vi "Module Top Level.vi"(8 "error in":errorcluster, 11 "Chassis3FPGA":T1) -> (0 "error out":errorcluster)   [LabVIEW 2018, in "ARINC.lvlib"]
doc: "This is the top level VI for this module. It uses a queue for communications and is stopped user a user event. The general architecture is similar to a simple queued message handler.\n\nThe VIs associated with this module are organized in a LabVIEW Library."
uses:
  ARINC.lvlib
  FPGA/Chassis3FPGARef.ctl
  Private Controls/Host Comms Data.ctl
  Private Controls/Module Data.ctl
  Private Controls/Module Action.ctl
  <vilib>/Utility/error.llb/Error Cluster From Error Code.vi
  <vilib>/rvi/errors/niLvFpgaAdjustHostInterfaceError.vi
  <vilib>/rvi/interface/nirviMethod/nirviMethod.xnode
  <vilib>/rvi/interface/nirviReadWriteControl/nirviReadWriteControl.xnode
  RT-UDP Writer/UDP Writer.lvlib
  <vilib>/FPGAPlugInAG/Dynamic/niLvFpga_AcknowledgeIrq_Dynamic.vi
  NiFpgaLv.dll
  <vilib>/rvi/interface/Simulation/niFpgaSimulationCallBeginRW.vi
  <vilib>/FPGAPlugInAG/Dynamic/niLvFpga_StartFifo_Dynamic.vi
  <vilib>/rvi/errors/niLvFpgaMergeErrorWithErrorCode.vi
panel:
  out "Data":u32[](array[numeric])
  # "ARINC"
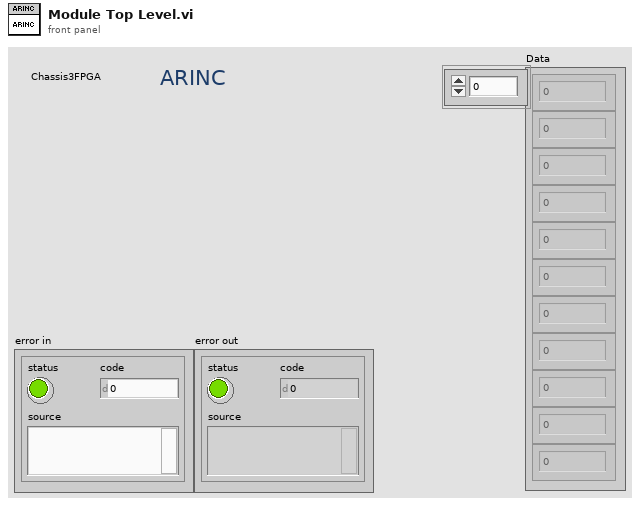
[diagram p1: front panel]
types:
  T1 = typedef "Chassis3FPGARef.ctl" = refnum<k20>
  T2 = typedef "ARINC.lvlib/Host Comms Data.ctl" = cluster{"Connected?":bool, "Arinc Data":sgl[]}
  T3 = typedef "ARINC.lvlib/Module Data.ctl" = cluster{"Data":variant, "Action":T4}
  T4 = typedef "ARINC.lvlib/Module Action.ctl" = enum16{"Init", "Write(Tx)", "Read(Rx)", "Error"}
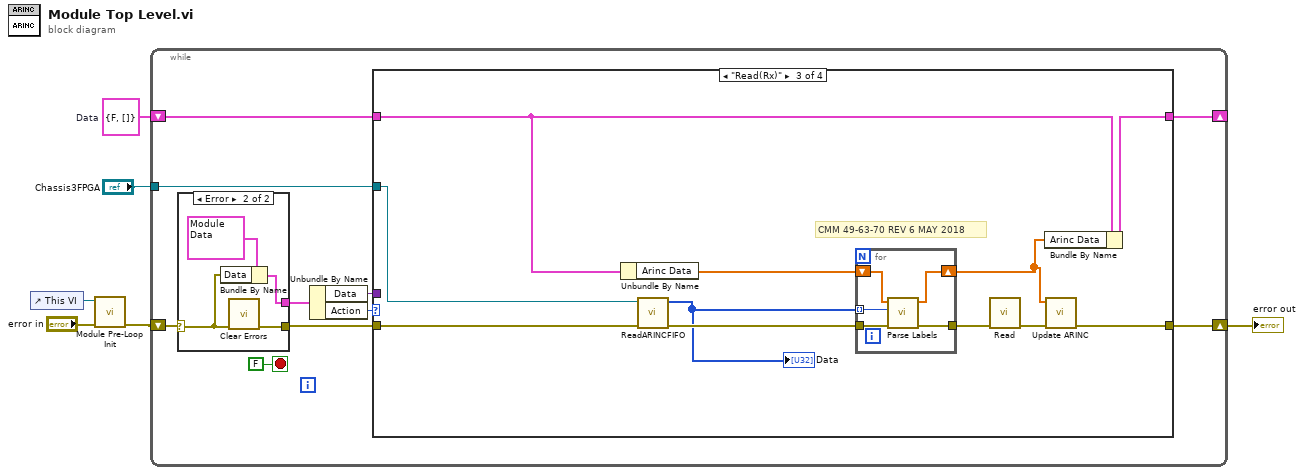
[diagram p0: block diagram]
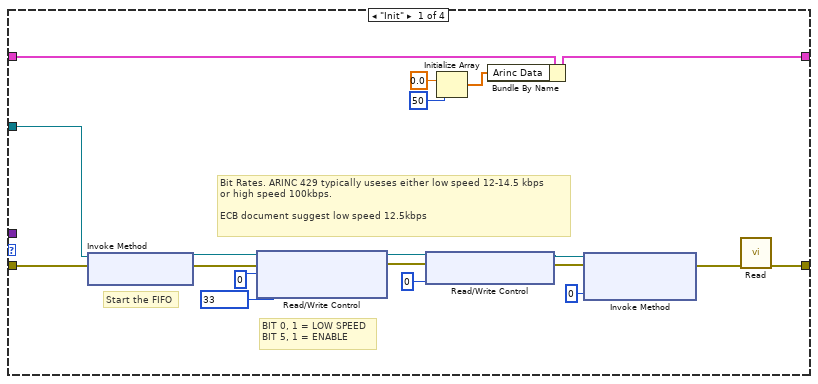
[diagram p2: hidden frame]
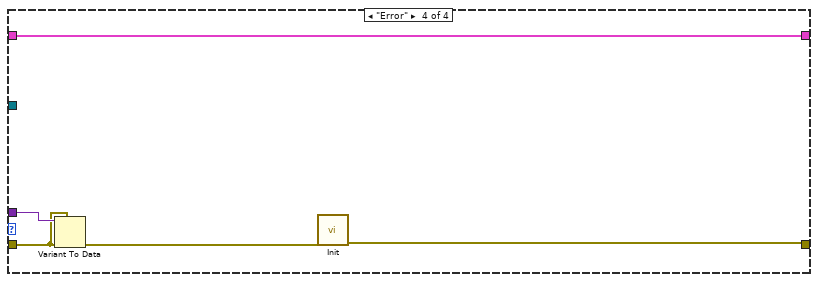
[diagram p4: hidden frame]
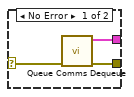
[diagram p5: hidden frame]
diagram:
  w3 = T2 {"Connected?"=FALSE, "Arinc Data"=[]}  # Data
  n1 = control-ref of="This VI"() -> (w6:refnum<vi>)
  n2 = call "Module Pre-Loop Init.vi"("error in (no error)"="error in", "Top Level VI Ref in"=w6) -> ("error out"=w2:errorcluster)  [unwired: 9 in]
  n3 = while {
    shift-right: [w12] -> w4
    shift-left: w2 -> [w11]
    shift-right: [w10] -> _
    shift-left: w3 -> [w9]
    tunnel: "Chassis3FPGA" -> [w7]
    stop <- FALSE stop-if-true
    n4 = case shown="Error" w11 {
      selector: w11 -> [w60 w63]
      tunnel: [w61 w64] -> w16
      tunnel: [w59 w62] -> w13
      frame No Error {
        n5 = call "Queue Comms Dequeue.vi"("error in (no error)"=w60) -> ("error out"=w59:errorcluster, "element"=w61:T3)  [unwired: 9 in]
      }
      frame Error {
        n6 = Bundle By Name(cluster=T3 {"Data"=variant, "Action"=enum."Error"} ("element"), "Data"=w63) -> (w64:T3)
        n7 = call <vilib>:"Clear Errors.vi"("error in (no error)"=w63) -> ("error out"=w62:errorcluster)  [unwired: 5 in, 1 out]
      }
    }
    n8 = Unbundle By Name(w16) -> ("Data"=w14:variant, "Action"=w15:T4)
    n9 = case shown="\"Read(Rx)\"" w15 {
      tunnel: w14 -> [_ _ _ w58]
      tunnel: w13 -> [w20 w37 w39 w57]
      tunnel: [w24 w37 w41 w55] -> w12
      tunnel: [w34 w36 w46 w54] -> w10
      tunnel: w9 -> [w35 w36 w48 w54]
      tunnel: w7 -> [w19 _ w38 _]
      frame "Init" {
        # "Bit Rates. ARINC 429 typically useses either low speed 12-14.5 kbps\nor high speed 100kbps.\n\nECB document suggest low speed 12.5kbps"
        # "BIT 0, 1 = LOW SPEED\nBIT 5, 1 = ENABLE"
        # "Start the FIFO"
        n10 = xnode "Invoke Method"("FPGA VI Reference In"=w19, "error in"=w20) -> ("FPGA VI Reference Out"=w17:T1, "error out"=w18:errorcluster)
        n11 = xnode "Read/Write Control"("FPGA VI Reference In"=w17, "error in"=w18, "Rx Channel Number"=u8 0, "Rx Config Data (RCR)"=u16 33) -> ("FPGA VI Reference Out"=w26:T1, "error out"=w25:errorcluster)
        n12 = xnode "Read/Write Control"("FPGA VI Reference In"=w26, "error in"=w25, "Tx Config Data (TCR)"=u16 0) -> ("FPGA VI Reference Out"=w23:T1, "error out"=w22:errorcluster)
        n13 = Initialize Array(sgl 0.0 ("element"), 50 ("dimension size")) -> (w33:sgl[])
        n14 = Bundle By Name(cluster=w35, "Arinc Data"=w33) -> (w34:T2)
        n15 = xnode "Invoke Method"("FPGA VI Reference In"=w23, "error in"=w22, "IRQ Number(s)"=0) -> ("error out"=w21:errorcluster)  [unwired: 1 out]
        n16 = call "Read.vi"("error in"=w21) -> ("error out"=w24:errorcluster)  [unwired: 10 in]
      }
      frame "Write(Tx)" {
      }
      frame "Read(Rx)" {
        # "CMM 49-63-70 REV 6 MAY 2018"
        n17 = Unbundle By Name(w48) -> ("Arinc Data"=w47:sgl[])
        n18 = call "ReadARINCFIFO.vi"("error in"=w39, "Refnum in"=w38) -> ("error out"=w44:errorcluster, "Data"=w43:u32[])  [unwired: 8 in]
        "Data" <- w43
        n19 = for {
          shift-right: [w52] -> w40
          shift-left: w47 -> [w53]
          tunnel: w43 -> [w49] mode=indexing
          tunnel: w44 -> [w50]
          tunnel: [w51] -> w45
          n20 = call "Parse Labels.vi"("error in"=w50, "Mod8/Rx0"=w49, "Arinc In"=w53) -> ("error out"=w51:errorcluster, "Arinc Out"=w52:sgl[])  [unwired: 7 in]
        }
        n21 = call "Read.vi"("error in"=w45) -> ("error out"=w42:errorcluster)  [unwired: 10 in]
        n22 = Bundle By Name(cluster=w48, "Arinc Data"=w40) -> (w46:T2)
        n23 = call "Update ARINC.vi"("error in"=w42, "ARINC"=w40) -> ("error out"=w41:errorcluster)  [unwired: 9 in]
      }
      frame "Error" {
        n24 = Variant To Data(error in=w57, type=w57, Variant=w58) -> (error out=w56:errorcluster)  [unwired: 1 out]
        n25 = call "Init.vi"("error in"=w56) -> ("error out"=w55:errorcluster)  [unwired: 10 in]
      }
    }
  }
  "error out" <- w4
